vi "getTaskChannelClassPath.vi"(5 "stopMechanismType":T1) -> (3 "ITaskClassPath":path)   [LabVIEW 2023]
uses:
  stopMechanismType.ctl
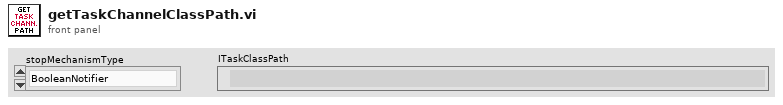
[diagram p1: front panel]
types:
  T1 = typedef "stopMechanismType.ctl" = enum16{"BooleanNotifier", "BooleanUE", "MsgUE", "MsgQueue"}
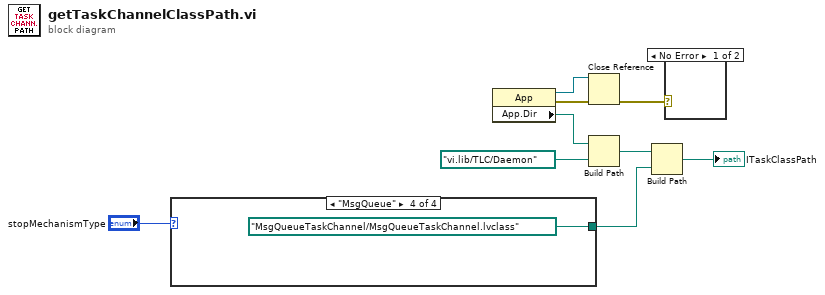
[diagram p0: block diagram]
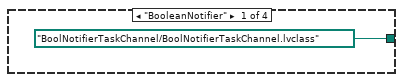
[diagram p3: hidden frame]
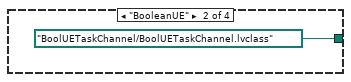
[diagram p4: hidden frame]
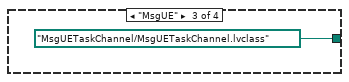
[diagram p5: hidden frame]
diagram:
  n1 = case shown="\"MsgQueue\"" "stopMechanismType" {
    tunnel: [path "BoolNotifierTaskChannel/BoolNotifierTaskChannel.lvclass" ("name or relative path") path "BoolUETaskChannel/BoolUETaskChannel.lvclass" ("name or relative path") path "MsgUETaskChannel/MsgUETaskChannel.lvclass" ("name or relative path") path "MsgQueueTaskChannel/MsgQueueTaskChannel.lvclass" ("name or relative path")] -> w4
    frame "BooleanNotifier" {
    }
    frame "BooleanUE" {
    }
    frame "MsgUE" {
    }
    frame "MsgQueue" {
    }
  }
  n2 = property class="App"() -> (reference out=w8:refnum<vi>, error out=w9:errorcluster, "App.Dir"=w7:path)  [unwired: 2 in]
  n3 = Close Reference(reference=w8, error in (no error)=w9) -> (error out=w1:errorcluster)
  n4 = Build Path(base path=w7, name or relative path=path "vi.lib/TLC/Daemon") -> (appended path=w3:path)
  n5 = Build Path(base path=w3, name or relative path=w4) -> (appended path=→"ITaskClassPath":path)
  n6 = case shown="No Error" w1 {
    frame No Error {
    }
    frame Error {
    }
  }
